vi "helper-log-parse-ntr.vi"(10 "output cluster":T1 {"clk" format="%#.3f"}) -> (2 "NTR Status":string, 3 "update?":bool)   [LabVIEW 2024]
uses:
  controls/typeEngineLogCluster.ctl
  controls/type.StepFunction.ctl
  controls/enum-ntr-io-format.ctl
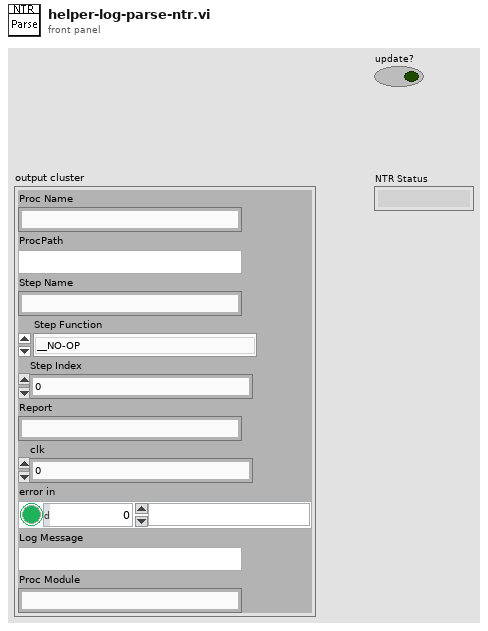
[diagram p1: front panel]
types:
  T1 = typedef "typeEngineLogCluster.ctl" = cluster{"Proc Name":string, "ProcPath":string, "Step Name":string, "Step Function":T2, "Step Index":i32, "Report":string, "clk":dbl, "error in":errorcluster, "Log Message":string, "Proc Module":string}
  T2 = typedef "type.StepFunction.ctl" = enum16{"__NO-OP", "_DELAY_LOAD", "_DELAY_COMPARE", "_JUMP", "_COMPLETE", "_COMPARE", "_LOG_MESSAGE", "_LOG_LAST_REPORT", "_SCHEDULE", "_SCHED_DAILY", "CLK_COMPARE", "PROC_START", "PROC_STOP", "PROC_LOAD", "PROC_COMPLETION_CHECK", "PROC_COMPLETION_LOAD", "_IO_READ", "_IO_READ_MANY", "_IO_WRITE", "_IO_WRITE_BY_REG", "_IO_GET_OUTPUT", "_OCS_CHECK", "_OCS_RECORD", "_GET_RH", "_GET_ACC_UV", "_GET_WD", "_GET_WS", "_REC_DELETE", "_REC_MOVE", "_REC_COPY", "_IRR_CHECK", "UNIT_CHECK", "UNIT_SAMPLE", "UNIT_DOSE"}
  T3 = typedef "enum-ntr-io-format.ctl" = enum16{"UN_VLV%d", "UN_PMP%d", "UN_WL%d", "UN_PH", "UN_EC", "UN_ORP", "UN_WT", "UN_PH2", "UN_ALFA1", "UN_BETA1", "UN_ALFA2", "UN_BETA2", "UN_ACID", "UN_BASE", "UN_WATER", "UN_ORPMIX"}
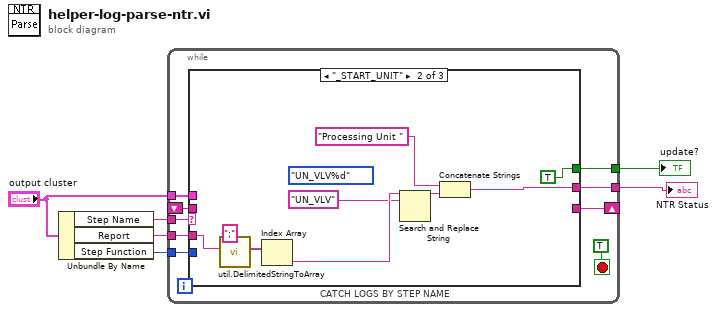
[diagram p0: block diagram]
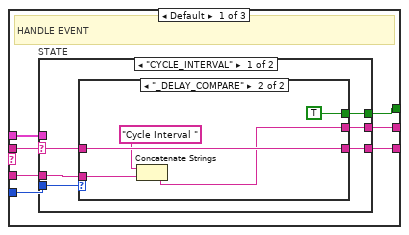
[diagram p2: hidden frame]
diagram:
  n1 = Unbundle By Name("output cluster") -> ("Step Name"=w2:string, "Report"=w3:string, "Step Function"=w4:T2)
  n2 = while {
    tunnel: w2 -> [w15]
    tunnel: "output cluster" -> [w14]
    tunnel: w3 -> [w13]
    shift-right: [w12] -> _
    shift-left: _ -> [w11]
    tunnel: w4 -> [w10]
    tunnel: [w8] -> w5
    tunnel: [w7] -> w6
    stop <- TRUE stop-if-true
    n3 = case "CATCH LOGS BY STEP NAME" shown="\"_START_UNIT\"" w15 {
      selector: w15 -> [_ _ w43]
      tunnel: w14 -> [w22 _ _]
      tunnel: w13 -> [w20 w42 _]
      tunnel: [w19 _ w43] -> w12
      tunnel: w11 -> [w18 _ _]
      tunnel: w10 -> [w21 _ _]
      tunnel: [w17 w36 _] -> w8
      tunnel: [w16 TRUE _] -> w7
      frame Default {
        # "HANDLE EVENT"
        n4 = case "STATE" shown="\"CYCLE_INTERVAL\"" w18 {
          selector: w18 -> [w25 _]
          tunnel: w22 -> [_ _]
          tunnel: w21 -> [w27 _]
          tunnel: w20 -> [w28 _]
          tunnel: [w26 _] -> w19
          tunnel: [w24 _] -> w17
          tunnel: [w23 _] -> w16
          frame "CYCLE_INTERVAL" {
            n5 = case shown="\"_DELAY_COMPARE\"" w27 {
              tunnel: w28 -> [_ w32]
              tunnel: [_ w33] -> w26
              tunnel: w25 -> [_ w33]
              tunnel: [_ w30] -> w24
              tunnel: [_ TRUE] -> w23
              frame Default {
              }
              frame "_DELAY_COMPARE" {
                n6 = Concatenate Strings("Cycle Interval " ("string"), w32) -> (w30:string)
              }
            }
          }
          frame Default {
          }
        }
      }
      frame "_START_UNIT" {
        (unwired) enum-ntr-io-format."UN_VLV%d"
        n7 = call "util.DelimitedStringToArray.vi"("delimiter (,)"=";", "delimitaed string"=w42) -> ("array out"=w40:string[])  [unwired: 9 in]
        n8 = Index Array(array=w40) -> (element=w39:string)  [unwired: 1 in]
        n9 = Search and Replace String(input string=w39, search string="UN_VLV") -> (result string=w37:string)  [unwired: 6 in, 3 out]
        n10 = Concatenate Strings("Processing Unit " ("string"), w37) -> (w36:string)
      }
      frame "CYCLE_INTERVAL" {
        # "CATCH CYCLE INTERVAL EVENT"
      }
    }
  }
  "update?" <- w6
  "NTR Status" <- w5
